vi "Init Top Level Tasks.vi"(8 "error in (no error)":errorcluster, 11 "VolatusCoreTask in":refnum<class "VolatusCoreTask.lvclass">) -> (0 "error out":errorcluster, 2 "Top Level Tasks":refnum<class "Task.lvclass">[](array[class]), 3 "VolatusCoreTask out":refnum<class "VolatusCoreTask.lvclass">)   [LabVIEW 2020, in "Volatus.lvlib" / "VolatusCoreTask.lvclass"]
uses:
  VolatusCoreTask.lvclass
  VolatusCoreTask.lvclass/VolatusCoreTask.ctl
  App/App.lvclass
  Task/Task.lvclass
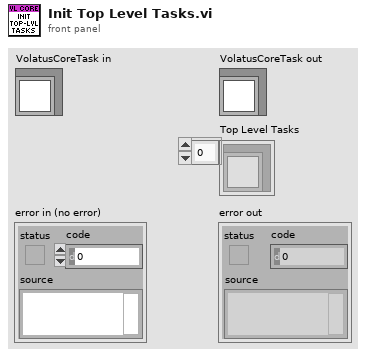
[diagram p1: front panel]
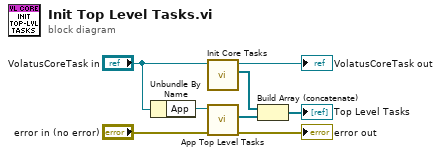
[diagram p0: block diagram]
diagram:
  n1 = Unbundle By Name("VolatusCoreTask in") -> ("App"=w6:refnum<class "App.lvclass">)
  n2 = call "Init Core Tasks.vi"("VolatusCoreTask in"="VolatusCoreTask in") -> ("Core Tasks"=w4:refnum<class "Task.lvclass">[], "VolatusCoreTask out"=→"VolatusCoreTask out":refnum<class "VolatusCoreTask.lvclass">)  [unwired: 8 in, 1 out]
  n3 = call-dynamic "App Top Level Tasks.vi"("error in (no error)"="error in (no error)", "App in"=w6) -> ("error out"=→"error out":errorcluster, "Top Level Tasks"=w3:refnum<class "Task.lvclass">[])  [unwired: 8 in]
  n4 = Build Array (concatenate)(w4, w3) -> (→"Top Level Tasks":refnum<class "Task.lvclass">[])
